vi "REPORT_DATES_delete_ID_column.vi"(11 "REPORT_DATES_all_info":T1) -> (3 "REPORT_DATES_all_info_ID_deleted":T1)   [LabVIEW 2019]
uses:
  typedef/REPORT_DATES_all_info.ctl
  typedef/REPORT_DATES_statuses.ctl
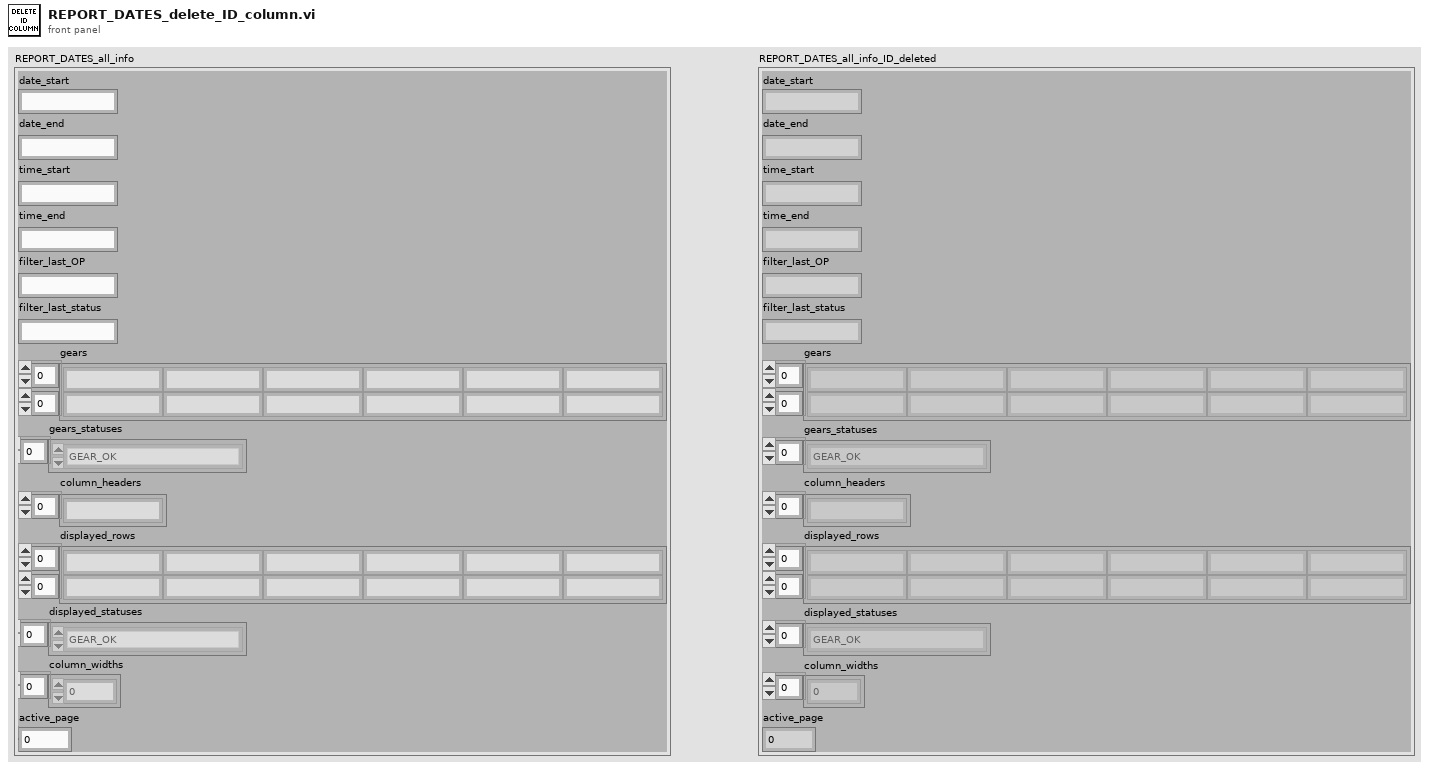
[diagram p1: front panel]
types:
  T1 = typedef "REPORT_DATES_all_info.ctl" = cluster{"date_start":string, "date_end":string, "time_start":string, "time_end":string, "filter_last_OP":string, "filter_last_status":string, "gears":string[][], "gears_statuses":T2[], "column_headers":string[], "displayed_rows":string[][], "displayed_statuses":T2[], "column_widths":i16[], "active_page":i32}
  T2 = typedef "REPORT_DATES_statuses.ctl" = enum16{"GEAR_OK", "GEAR_NOK", "GEAR_interrupted", "GEAR_in_operation", "GEAR_unexpected"}
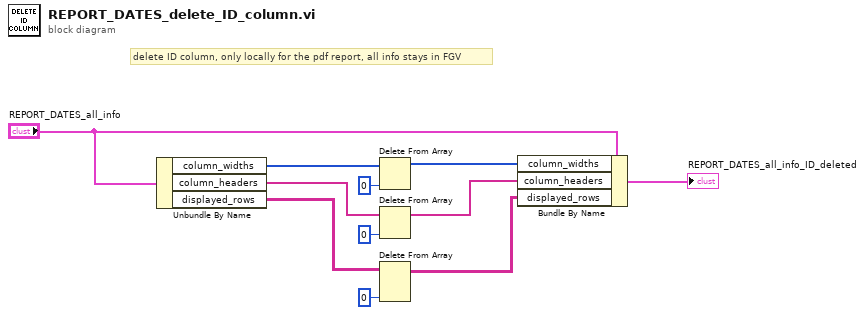
[diagram p0: block diagram]
diagram:
  # "delete ID column, only locally for the pdf report, all info stays in FGV"
  n1 = Unbundle By Name("REPORT_DATES_all_info") -> ("column_widths"=w11:i16[], "column_headers"=w10:string[], "displayed_rows"=w9:string[][])
  n2 = Delete From Array(array=w11, index=0) -> (array with subset deleted=w3:i16[])  [unwired: 1 in, 1 out]
  n3 = Delete From Array(array=w10, index=0) -> (array with subset deleted=w2:string[])  [unwired: 1 in, 1 out]
  n4 = Delete From Array(array=w9, index (col)=0 ("disabled index (col)")) -> (array with subset deleted=w1:string[][])  [unwired: 2 in, 1 out]
  n5 = Bundle By Name(cluster="REPORT_DATES_all_info", "column_widths"=w3, "column_headers"=w2, "displayed_rows"=w1) -> (→"REPORT_DATES_all_info_ID_deleted":T1)
